vi "相机4初始化.vi"() -> (1 "Session Out":T2, 2 "Image":T1, 3 "相机状态":bool, 4 "error out":errorcluster)   [LabVIEW 2014]
uses:
  <vilib>/userdefined/High Color/IMAQdx.ctl
  <vilib>/vision/Image Controls.llb/IMAQ Image.ctl
  Controls/MsgAction.ctl
  Global.vi
  <vilib>/vision/driver/NI_Vision_Acquisition_Software.lvlib
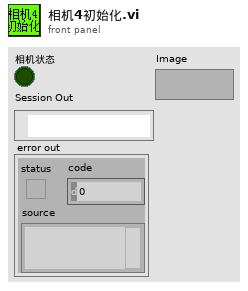
[diagram p1: front panel]
types:
  T1 = typedef "IMAQ Image.ctl" = refnum<image>
  T2 = typedef "IMAQdx.ctl" = refnum<k21>
  T3 = typedef "MsgAction.ctl" = enum16{"初始化", "添加消息", "区分结果添加消息", "清空消息", "获取消息"}
  T4 = typedef "OtherSpec.ctl" = cluster{"其它勾选类规格":T5, "其它数据类规格":T6, "相机名称":T7}
  T5 = typedef "其它勾选类规格.ctl" = cluster{"保存NG图片":bool, "保存OK图片":bool, "保存数据":bool, "连接远程数据库":bool, "开机默认开启锁附监控摄像头":bool, "开机默认开启全景监控摄像头":bool, "保存自动运行时监控视频":bool, "自动页面显示拍照实时按钮":bool, "放螺杆坐标采用当前拍Mark点计算数据":bool}
  T6 = typedef "其他数据类规格.ctl" = cluster{"相机1像素-毫米换算系数":dbl, "相机2像素-毫米换算系数":dbl, "相机3像素-毫米换算系数":dbl, "相机4像素-毫米换算系数":dbl, "D盘剩余空间预警(G)":dbl, "视频最长录制时间(秒)":dbl}
  T7 = typedef "相机名称品牌使用状态.ctl" = cluster{"相机1名称":T2, "相机2名称":T2, "相机3名称":T2, "相机4名称":T2, "Cam1启用":bool, "Cam2启用":bool, "Cam3启用":bool, "Cam4启用":bool, "Basler1":bool, "Basler2":bool, "Basler3":bool, "Basler4":bool}
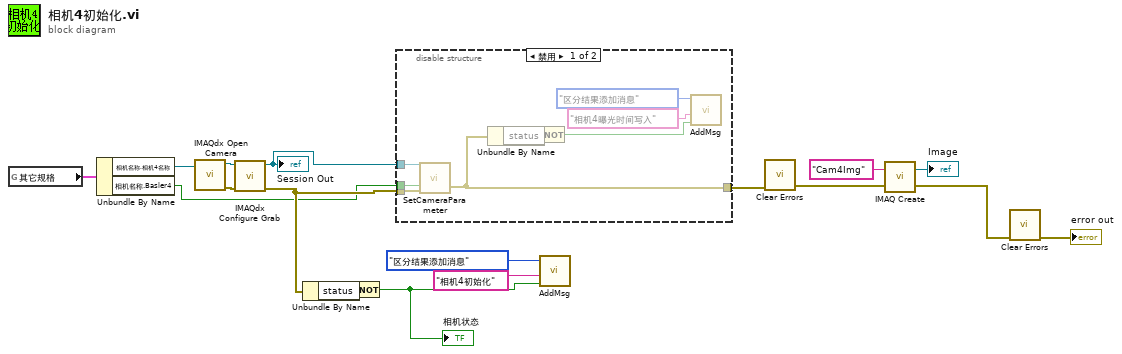
[diagram p0: block diagram]
diagram:
  n1 = global read "Global.vi" "其它规格"() -> (w10:T4)
  n2 = Unbundle By Name(w10) -> ("相机名称.相机4名称"=w11:T2, "相机名称.Basler4"=w1:bool)
  n3 = call <vilib>:"IMAQdx Open Camera.vi"("Session In"=w11) -> ("error out"=w16:errorcluster, "Session Out"=w15:T2)  [unwired: 9 in]
  n4 = call <vilib>:"IMAQdx Configure Grab.vi"("error in"=w16, "Session In"=w15) -> ("error out"=w5:errorcluster, "Session Out"=w4:T2)  [unwired: 8 in]
  "Session Out" <- w4
  n5 = Unbundle By Name(w5) -> ("status"=w12:bool)
  n6 = Not(x=w12) -> (.not. x?=w17:bool)
  "相机状态" <- w17
  n7 = disable-structure shown="禁用" {
    disable-tunnel: w5 -> [w21 w26]
    disable-tunnel: w4 -> [w20 _]
    disable-tunnel: [w19 w26] -> w2
    disable-tunnel: w1 -> [w18 _]
    frame Disabled {
      n8 = call "SetCameraParameter.vi"("error in"=w21, "相机品牌为Basler?"=w18, "Session In"=w20) -> ("error out"=w19:errorcluster)  [unwired: 1 in, 1 out]
      n9 = Unbundle By Name(w19) -> ("status"=w25:bool)
      n10 = Not(x=w25) -> (.not. x?=w22:bool)
      n11 = call "AddMsg.vi"("Result"=w22, "添加消息"="相机4曝光时间写入" ("消息显示"), "消息Action"=MsgAction."区分结果添加消息") -> ()  [unwired: 1 in, 1 out]
    }
    frame Enabled {
    }
  }
  n12 = call "AddMsg.vi"("Result"=w17, "添加消息"="相机4初始化" ("消息显示"), "消息Action"=MsgAction."区分结果添加消息") -> ()  [unwired: 1 in, 1 out]
  n13 = call <vilib>:"Clear Errors.vi"("error in (no error)"=w2) -> ("error out"=w6:errorcluster)  [unwired: 5 in, 1 out]
  n14 = call "IMAQ Create"("Image Name"="Cam4Img", "error in (no error)"=w6) -> ("New Image"=→"Image":T1, "error out"=w8:errorcluster)  [unwired: 3 in]
  n15 = call <vilib>:"Clear Errors.vi"("error in (no error)"=w8) -> ("error out"=→"error out":errorcluster)  [unwired: 5 in, 1 out]
